vi "Read Shared Variables - SuNLaMP Relay Outputs.vi"(9 "channel errors in (no errors)":errorcluster[](array[cluster])) -> (1 "channel errors out":errorcluster[](array[cluster]), 2 "data":dbl[](array[numeric]), 3 "UUIDs":string[](array[string])=["Flow Rate [g/s]", "Density [g/cm^3]", "Return Filter dP [psid]", "Outlet Filter and Flowmeter dp [psid]", "Cooler dP [psid]", "Cooler CO2 In [F]", "Cooler CO2 Out [F]", "Pump Frequency [%]", "Recirc Valve Open [%]"])   [LabVIEW 2020]
uses:
  <vilib>/Utility/error.llb/Error Cluster From Error Code.vi
  <vilib>/ErrorRing/Error Ring.xnode
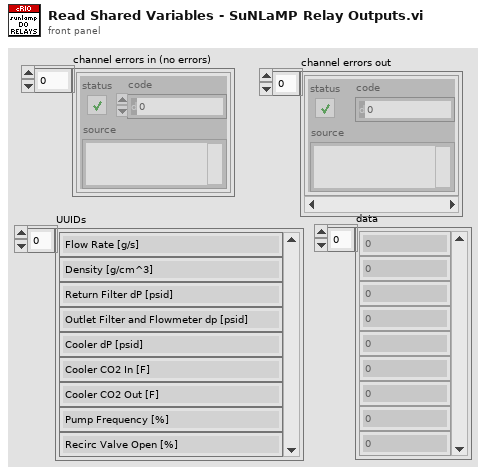
[diagram p1: front panel]
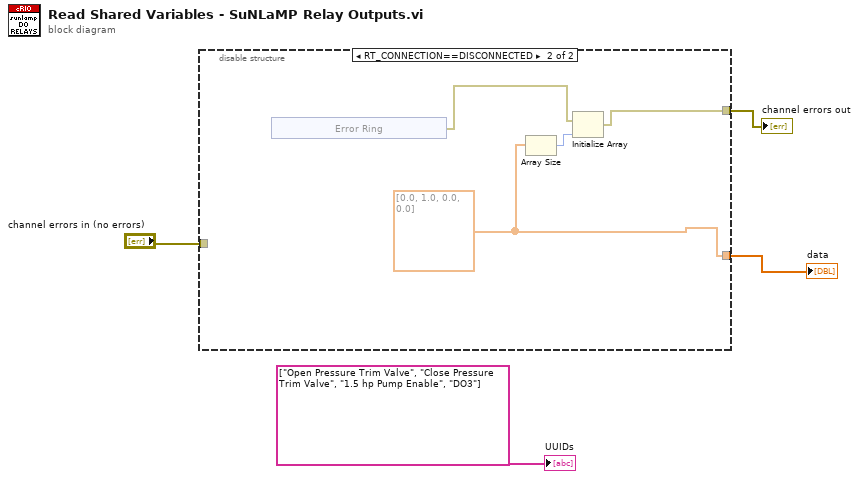
[diagram p0: block diagram]
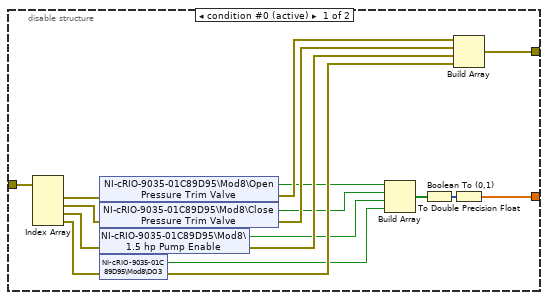
[diagram p2: hidden frame]
diagram:
  n1 = disable-structure shown="RT_CONNECTION==DISCONNECTED" {
    disable-tunnel: [w13 w23] -> w3
    disable-tunnel: "channel errors in (no errors)" -> [w12 _]
    disable-tunnel: [w5 w24] -> w1
    frame condition #0 (active) {
      n2 = Index Array(array=w12) -> (element #1=w11:errorcluster, element #2=w10:errorcluster, element #3=w9:errorcluster, element #4=w8:errorcluster)  [unwired: 4 in]
      n3 = shared-variable "NI-cRIO-9035-01C89D95\\Mod8\\Open Pressure Trim Valve"(error in=w11) -> (w14:bool, error out=w18:errorcluster)
      n4 = shared-variable "NI-cRIO-9035-01C89D95\\Mod8\\Close Pressure Trim Valve"(error in=w10) -> (w15:bool, error out=w19:errorcluster)
      n5 = shared-variable "NI-cRIO-9035-01C89D95\\Mod8\\1.5 hp Pump Enable"(error in=w9) -> (w16:bool, error out=w20:errorcluster)
      n6 = shared-variable "NI-cRIO-9035-01C89D95\\Mod8\\DO3"(error in=w8) -> (w17:bool, error out=w21:errorcluster)
      n7 = Build Array(w14, w15, w16, w17) -> (w6:bool[])
      n8 = Boolean To (0,1)(Boolean=w6) -> (0, 1=w7:i16[])
      n9 = Build Array(w18, w19, w20, w21) -> (w13:errorcluster[])
      n10 = To Double Precision Float(number=w7) -> (double precision float=w5:dbl[])
    }
    frame condition #1 {
      w24 = dbl[] [0.0, 1.0, 0.0, 0.0] ("data")
      n11 = xnode "Error Ring"() -> ("error out"=w22:errorcluster)
      n12 = Array Size(array=w24) -> (size(s)=w25:i32)
      n13 = Initialize Array(w22, w25) -> (w23:errorcluster[])
    }
  }
  "data" <- w1
  "channel errors out" <- w3
  "UUIDs" <- string[] ["Open Pressure Trim Valve", "Close Pressure Trim Valve", "1.5 hp Pump Enable", "DO3"]
